vi "Find Project VIs.vi"(7 "App Reference (This Application)":refnum<vi>, 8 "error in (no error)":errorcluster {"code" format="Error %.0f"}, 11 "LabVIEW Project Path":path) -> (0 "error out":errorcluster {"code" format="Error %.0f"}, 3 "Project VI Paths":path[](array[path]))   [LabVIEW 2023]
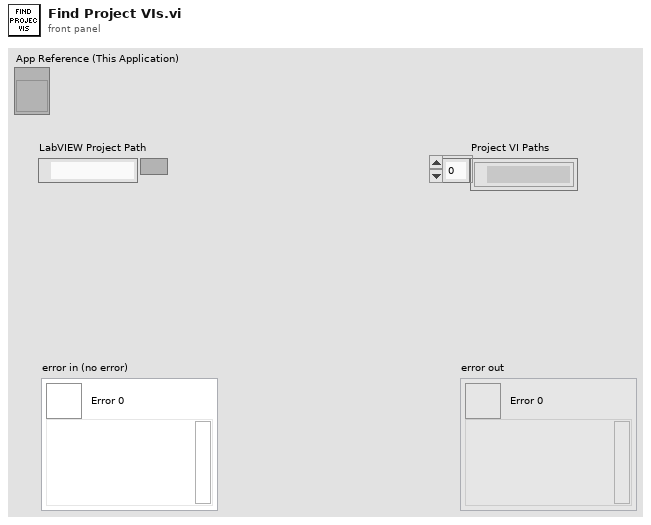
[diagram p1: front panel]
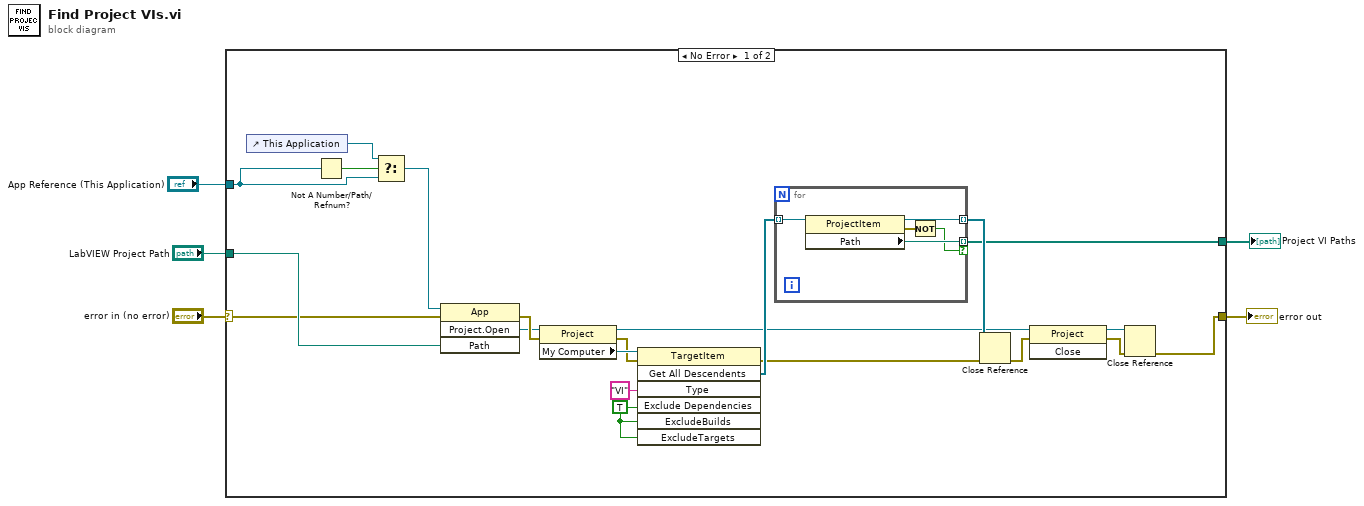
[diagram p0: block diagram]
diagram:
  n1 = case shown="No Error" "error in (no error)" {
    selector: "error in (no error)" -> [w11 w32]
    tunnel: [w13 w32] -> w4
    tunnel: "LabVIEW Project Path" -> [w26 _]
    tunnel: [w12 _] -> w2
    tunnel: "App Reference (This Application)" -> [w8 _]
    frame No Error {
      w25 = TRUE ("ExcludeDependencies")
      n2 = control-ref of="This Application"() -> (w9:refnum<vi>)
      n3 = Not A Number/Path/Refnum?(number/path/refnum=w8) -> (NaN/Path/Refnum?=w10:bool)
      n4 = Select(t=w9, s=w10, f=w8) -> (s? t:f=w7:refnum<vi>)
      n5 = invoke class="App" method="Project.Open"(reference=w7, error in=w11, "Path"=w26) -> (error out=w23:errorcluster, "Project:Open"=w18:refnum<vi>)  [unwired: 1 in, 2 out]
      n6 = property class="Project"(reference=w18, error in=w23) -> (reference out=w17:refnum<vi>, error out=w21:errorcluster, "My Computer"=w22:refnum<vi>)
      n7 = invoke class="TargetItem" method="Get All Descendents"(reference=w22, error in=w21, "Type"="VI", "Exclude Dependencies"=w25, "ExcludeBuilds"=w25, "ExcludeTargets"=w25) -> (error out=w6:errorcluster, "All Descendents"=w20:refnum<vi>[])  [unwired: 1 in, 5 out]
      n8 = for {
        tunnel: w20 -> [w31] mode=indexing
        tunnel: [w28] -> w12 mode=indexing if=w27
        tunnel: [w29] -> w19 mode=indexing
        n9 = property class="ProjectItem"(reference=w31) -> (reference out=w29:refnum<vi>, error out=w30:errorcluster, "Path"=w28:path)  [unwired: 1 in]
        n10 = Not(x=w30) -> (.not. x?=w27:bool)
      }
      n11 = Close Reference(reference=w19, error in (no error)=w6) -> (error out=w16:errorcluster)
      n12 = invoke class="Project" method="Close"(reference=w17, error in=w16) -> (reference out=w14:refnum<vi>, error out=w15:errorcluster)  [unwired: 1 in, 1 out]
      n13 = Close Reference(reference=w14, error in (no error)=w15) -> (error out=w13:errorcluster)
    }
    frame Error {
    }
  }
  "error out" <- w4
  "Project VI Paths" <- w2
